vi "U8数组转变量.vi"(7 "Control输入":refnum<vi>, 8 "错误输入（无错误）":errorcluster, 11 "数组输入":u8[](array[numeric])) -> (0 "错误输出":errorcluster, 3 "数组输出":u8[](array[numeric]))   [LabVIEW 2016, in "斯坦道总磷.lvlib"]
uses:
  <vilib>/Utility/miscctls.llb/LVDateTimeRec.ctl
  <vilib>/Utility/Data Type/NI_Data Type.lvlib
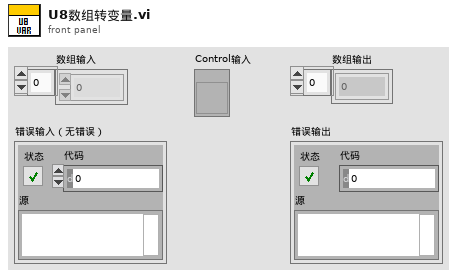
[diagram p1: front panel]
types:
  T1 = typedef "NI_Data Type.lvlib/Data Type.ctl" = enum8{"Invalid Type", "Void", "I8", "I16", "I32", "I64", "U8", "U16", "U32", "U64", "Single Float", "Double Float", "Extended Float", "Single Complex", "Double Complex", "Extended Complex", "Enum U8", "Enum U16", "Enum U32", "Enum U64", "Single Float With Unit", "Double Float With Unit", "Extended Float With Unit", "Single Complex with Unit", "Double Complex with Unit", "Extended Complex with Unit", "Boolean", "String", "Path", "Picture", "Tag", "Array", "Cluster", "Variant", "LV Variant", "Waveform", "Timestamp", "Digital Waveform", "Digital Data", "ExpressData", "Refnum", "External Data", "VI", "Poly VI", "LabVIEW Class Instance", "Fixed Point"}
  T2 = typedef "LVDateTimeRec.ctl" = cluster{"fractional second":dbl, "second":i32, "minute":i32, "hour":i32, "day of month":i32, "month":i32, "year":i32, "day of week":i32, "day of year":i32, "DST":i32}
  T3 = cluster{"标准值":sgl, "吸光值":sgl, "启用":bool, "数据时间":timestamp}
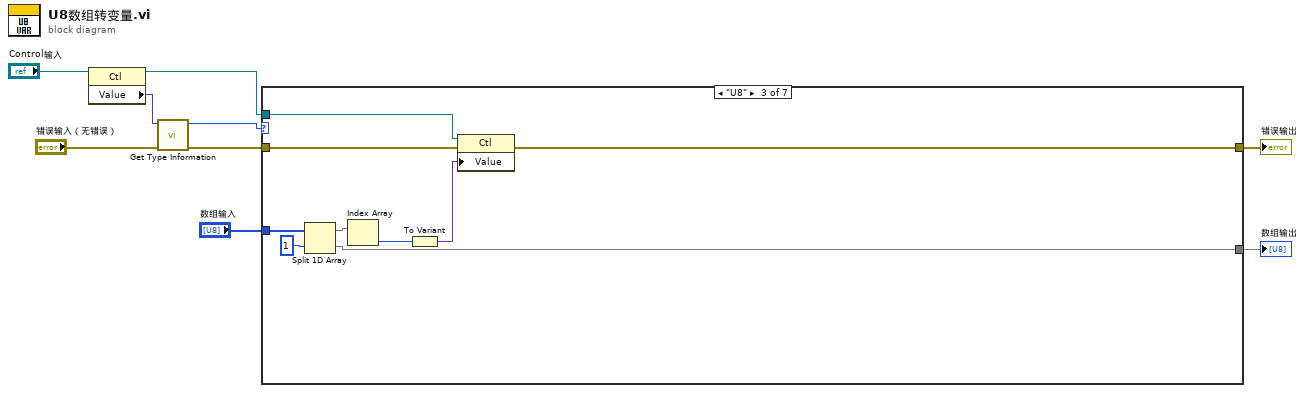
[diagram p0: block diagram]
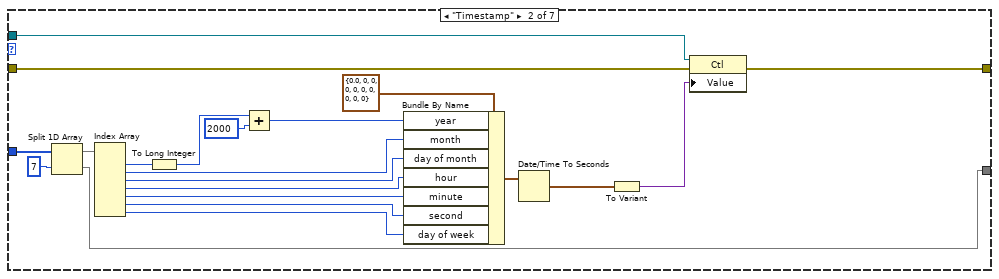
[diagram p3: hidden frame]
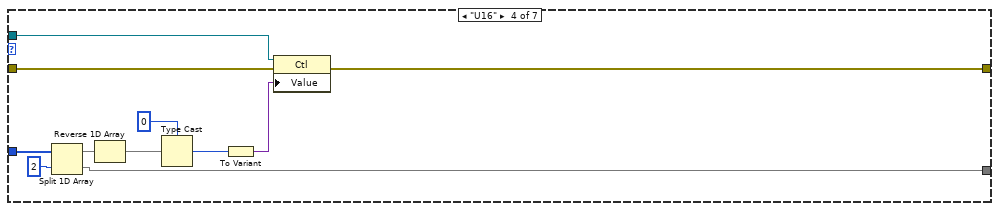
[diagram p4: hidden frame]
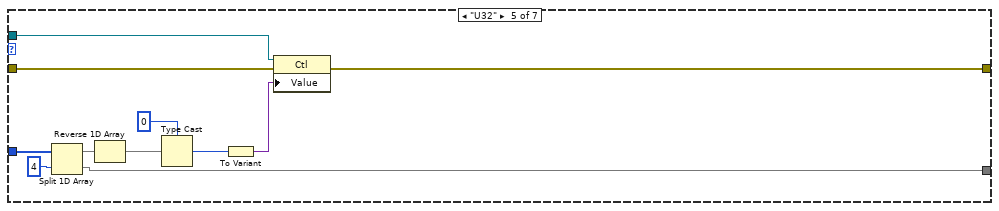
[diagram p5: hidden frame]
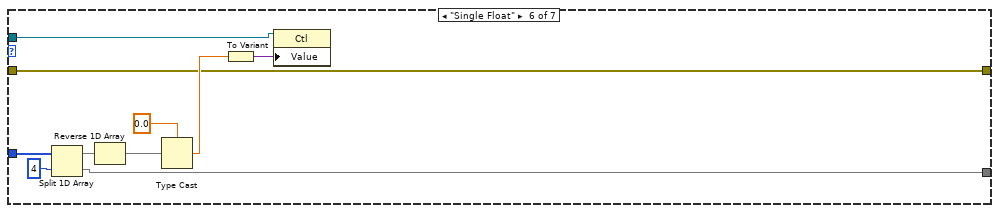
[diagram p6: hidden frame]
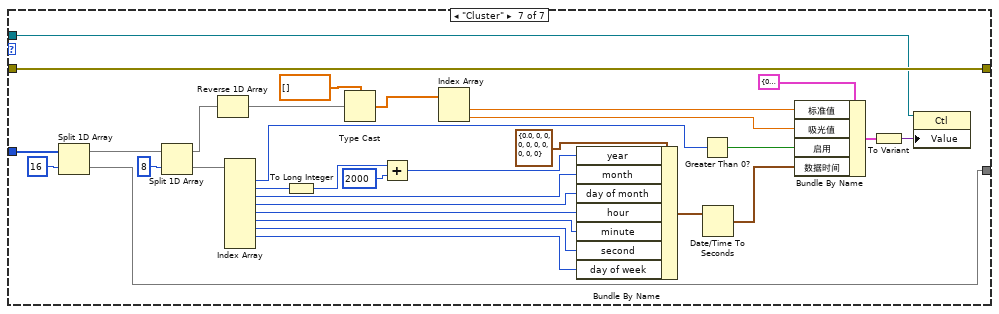
[diagram p7: hidden frame]
diagram:
  n1 = property class="Ctl"(reference="Control输入") -> (reference out=w9:refnum<vi>, "Value"=w8:variant)  [unwired: 1 in, 1 out]
  n2 = call <vilib>:"Get Type Information.vi"("error in (no error)"="错误输入（无错误）", "Variant"=w8) -> ("error out"=w3:errorcluster, "Type"=w2:T1)  [unwired: 5 in, 3 out]
  n3 = case shown="\"U8\"" w2 {
    tunnel: [_ w20 w38 w49 w60 w70 w102] -> w5
    tunnel: w3 -> [w10 w13 w34 w42 w53 w65 w101]
    tunnel: [w10 w12 w33 w41 w52 w65 w101] -> w4
    tunnel: "数组输入" -> [_ w30 w40 w51 w62 w72 w104]
    tunnel: w9 -> [_ w11 w32 w46 w56 w63 w99]
    frame "Invalid Type", Default {
    }
    frame "Timestamp" {
      n4 = Split 1D Array(array=w30, index=7 ("索引")) -> (first subarray=w28:u8[], second subarray=w20:u8[])
      n5 = Index Array(array=w28) -> (element #1=w19:u8, element #2=w27:u8, element #3=w26:u8, element #4=w25:u8, element #5=w24:u8, element #6=w23:u8, element #7=w22:u8)  [unwired: 7 in]
      n6 = To Long Integer(number=w19) -> (32bit integer=w18:i32)
      n7 = Add(x=w18, y=2000) -> (x+y=w17:i32)
      n8 = Bundle By Name(cluster=T2 {"fractional second"=0.0, "second"=0, "minute"=0, "hour"=0, "day of month"=0, "month"=0, "year"=0, "day of week"=0, "day of year"=0, "DST"=0} ("输入簇"), "year"=w17, "month"=w27, "day of month"=w26, "hour"=w25, "minute"=w24, "second"=w23, "day of week"=w22) -> (w21:T2)
      n9 = Date/Time To Seconds(2:w21) -> (0:w15:timestamp)  [unwired: 1 in]
      n10 = To Variant(anything=w15) -> (Variant=w14:variant)
      n11 = property class="Ctl"(reference=w11, error in=w13, "Value"=w14) -> (error out=w12:errorcluster)  [unwired: 1 out]
    }
    frame "U8" {
      n12 = Split 1D Array(array=w40, index=1 ("索引")) -> (first subarray=w37:u8[], second subarray=w38:u8[])
      n13 = Index Array(array=w37) -> (element=w36:u8)  [unwired: 1 in]
      n14 = To Variant(anything=w36) -> (Variant=w35:variant)
      n15 = property class="Ctl"(reference=w32, error in=w34, "Value"=w35) -> (error out=w33:errorcluster)  [unwired: 1 out]
    }
    frame "U16" {
      n16 = Split 1D Array(array=w51, index=2 ("索引")) -> (first subarray=w48:u8[], second subarray=w49:u8[])
      n17 = Reverse 1D Array(array=w48) -> (reversed array=w47:u8[])
      n18 = Type Cast(type=u16 0, x=w47) -> (*(type *) &x=w44:u16)
      n19 = To Variant(anything=w44) -> (Variant=w43:variant)
      n20 = property class="Ctl"(reference=w46, error in=w42, "Value"=w43) -> (error out=w41:errorcluster)  [unwired: 1 out]
    }
    frame "U32" {
      n21 = Split 1D Array(array=w62, index=4 ("索引")) -> (first subarray=w59:u8[], second subarray=w60:u8[])
      n22 = Reverse 1D Array(array=w59) -> (reversed array=w58:u8[])
      n23 = Type Cast(type=u32 0, x=w58) -> (*(type *) &x=w55:u32)
      n24 = To Variant(anything=w55) -> (Variant=w54:variant)
      n25 = property class="Ctl"(reference=w56, error in=w53, "Value"=w54) -> (error out=w52:errorcluster)  [unwired: 1 out]
    }
    frame "Single Float" {
      n26 = Split 1D Array(array=w72, index=4 ("索引")) -> (first subarray=w69:u8[], second subarray=w70:u8[])
      n27 = Reverse 1D Array(array=w69) -> (reversed array=w68:u8[])
      n28 = Type Cast(type=sgl 0.0, x=w68) -> (*(type *) &x=w66:sgl)
      n29 = To Variant(anything=w66) -> (Variant=w64:variant)
      n30 = property class="Ctl"(reference=w63, "Value"=w64) -> ()  [unwired: 1 in, 2 out]
    }
    frame "Cluster" {
      n31 = Split 1D Array(array=w104, index=16 ("索引")) -> (first subarray=w98:u8[], second subarray=w102:u8[])
      n32 = Split 1D Array(array=w98, index=8 ("索引")) -> (first subarray=w96:u8[], second subarray=w89:u8[])
      n33 = Reverse 1D Array(array=w96) -> (reversed array=w95:u8[])
      n34 = Index Array(array=w89) -> (element #1=w88:u8, element #2=w82:u8, element #3=w81:u8, element #4=w80:u8, element #5=w79:u8, element #6=w78:u8, element #7=w77:u8, element #8=w76:u8)  [unwired: 9 in, 1 out]
      n35 = To Long Integer(number=w82) -> (32bit integer=w85:i32)
      n36 = Type Cast(type=sgl[] [], x=w95) -> (*(type *) &x=w92:sgl[])
      n37 = Add(x=w85, y=2000) -> (x+y=w84:i32)
      n38 = Index Array(array=w92) -> (element #1=w91:sgl, element #2=w90:sgl)  [unwired: 2 in]
      n39 = Bundle By Name(cluster=T2 {"fractional second"=0.0, "second"=0, "minute"=0, "hour"=0, "day of month"=0, "month"=0, "year"=0, "day of week"=0, "day of year"=0, "DST"=0} ("输入簇"), "year"=w84, "month"=w81, "day of month"=w80, "hour"=w79, "minute"=w78, "second"=w77, "day of week"=w76) -> (w75:T2)
      n40 = Greater Than 0?(x=w88) -> (x > 0?=w87:bool)
      n41 = Date/Time To Seconds(2:w75) -> (0:w74:timestamp)  [unwired: 1 in]
      n42 = Bundle By Name(cluster=T3 {"标准值"=0.0, "吸光值"=0.0, "启用"=FALSE, "数据时间"=timestamp(0 s since 1904-01-01)} ("校准值一"), "标准值"=w91, "吸光值"=w90, "启用"=w87, "数据时间"=w74) -> (w73:T3)
      n43 = To Variant(anything=w73) -> (Variant=w100:variant)
      n44 = property class="Ctl"(reference=w99, "Value"=w100) -> ()  [unwired: 1 in, 2 out]
    }
  }
  "数组输出" <- w5
  "错误输出" <- w4
